vi "if flyback.vi"(5 "y#":dbl, 7 "x#":dbl, 9 "flyback step#":dbl, 10 "frame count":dbl) -> (3 "save?":bool, 4 "one frame #":dbl)   [LabVIEW 2015]
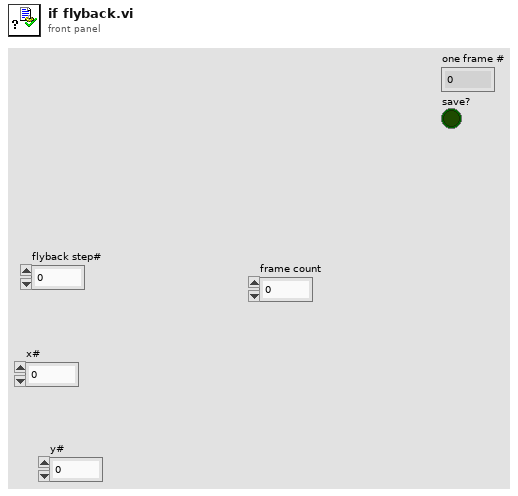
[diagram p1: front panel]
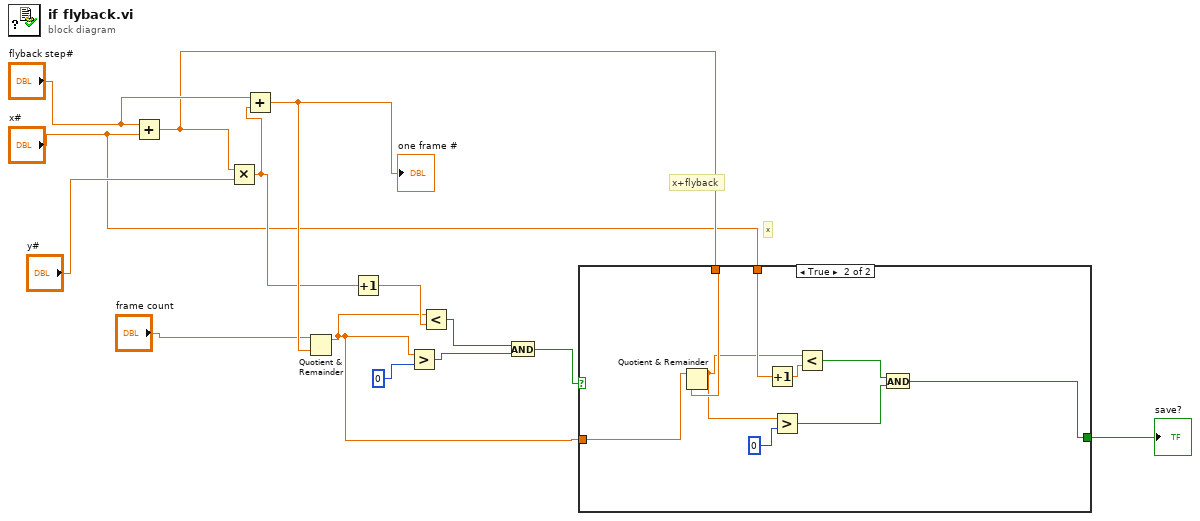
[diagram p0: block diagram]
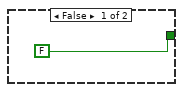
[diagram p2: hidden frame]
diagram:
  # "x"
  # "x+flyback"
  n1 = Add(x="flyback step#", y="x#") -> (x+y=w2:dbl)
  n2 = Multiply(x=w2, y="y#") -> (x*y=w10:dbl)
  n3 = Add(x="flyback step#", y=w10) -> (x+y=w13:dbl)
  "one frame #" <- w13
  n4 = Quotient & Remainder(x="frame count", y=w13) -> (x-y*floor(x/y)=w3:dbl)  [unwired: 1 out]
  n5 = Increment(x=w10) -> (x+1=w9:dbl)
  n6 = Greater?(x=w3, y=0) -> (0:w7:bool)
  n7 = Less?(x=w3, y=w9) -> (x < y?=w6:bool)
  n8 = And(x=w6, y=w7) -> (x .and. y?=w5:bool)
  n9 = case shown="True" w5 {
    tunnel: [FALSE w16] -> w4
    tunnel: w3 -> [_ w24]
    tunnel: w2 -> [_ w23]
    tunnel: "x#" -> [_ w22]
    frame False {
    }
    frame True {
      n10 = Quotient & Remainder(x=w24, y=w23) -> (x-y*floor(x/y)=w20:dbl)  [unwired: 1 out]
      n11 = Increment(x=w22) -> (x+1=w21:dbl)
      n12 = Greater?(x=w20, y=0) -> (0:w17:bool)
      n13 = Less?(x=w20, y=w21) -> (x < y?=w18:bool)
      n14 = And(x=w18, y=w17) -> (x .and. y?=w16:bool)
    }
  }
  "save?" <- w4
